vi "PreferenceFolder.vi"() -> (0 "error out":errorcluster, 1 "Colors":u32[](array[numeric]), 2 "FontSize":u8, 3 "pythonCodes":path[](array[path]), 4 "SSH Logins":T3(array[cluster]), 5 "Examples":path, 6 "Pis":T2(array[cluster]), 7 "Everything":T1={"python"="", "arduino CLI"=path "", "pythonCodes"=[], "FontSize"=0, "Text Colors"={"Quote"=46086, "function"=239, "Python"=11817216, "Comment"=15665920, "Triple Quote"=9306312, "Text"=0}, "SSH Logins"=[], "packet size"=32})   [LabVIEW 2024]
uses:
  Preferences.ctl
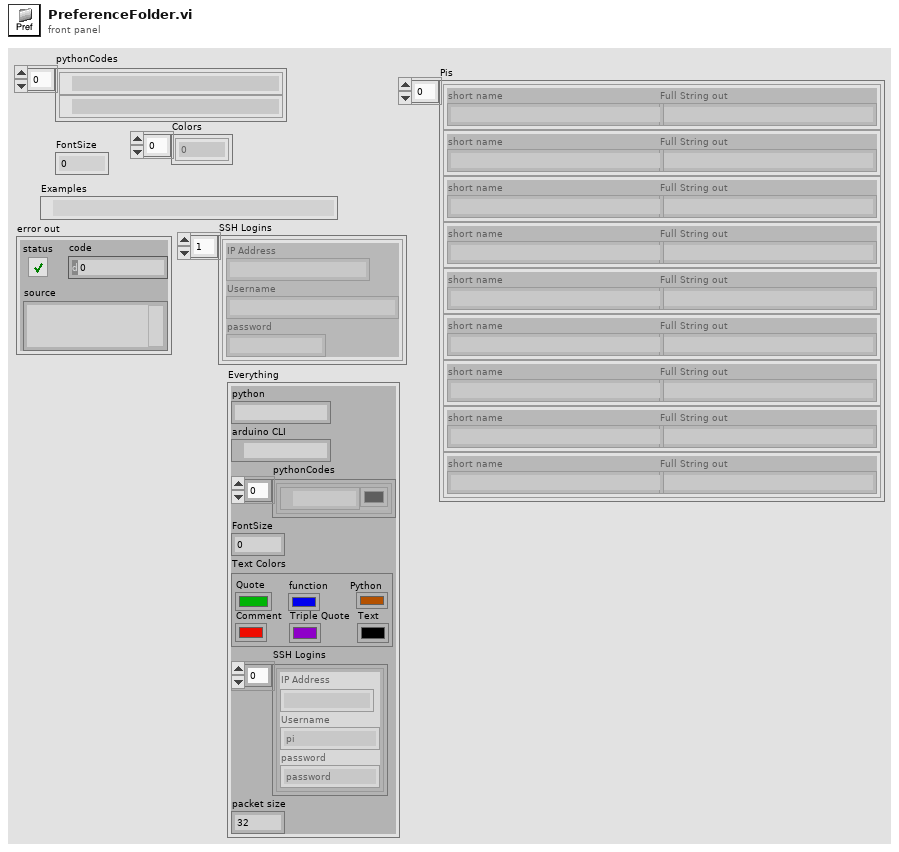
[diagram p1: front panel]
types:
  T1 = typedef "Preferences.ctl" = cluster{"python":string, "arduino CLI":path, "pythonCodes":cluster{"pythonCode":path, "Color":u32}[], "FontSize":u8, "Text Colors":cluster{"Quote":u32, "function":u32, "Python":u32, "Comment":u32, "Triple Quote":u32, "Text":u32}, "SSH Logins":cluster{"IP Address":string, "Username":string, "password":string}[], "packet size":u8}
  T2 = cluster{"short name":string, "Full String out":string}[]
  T3 = cluster{"IP Address":string, "Username":string, "password":string}[]
  T4 = cluster{"short name":string, "Full String out":string}
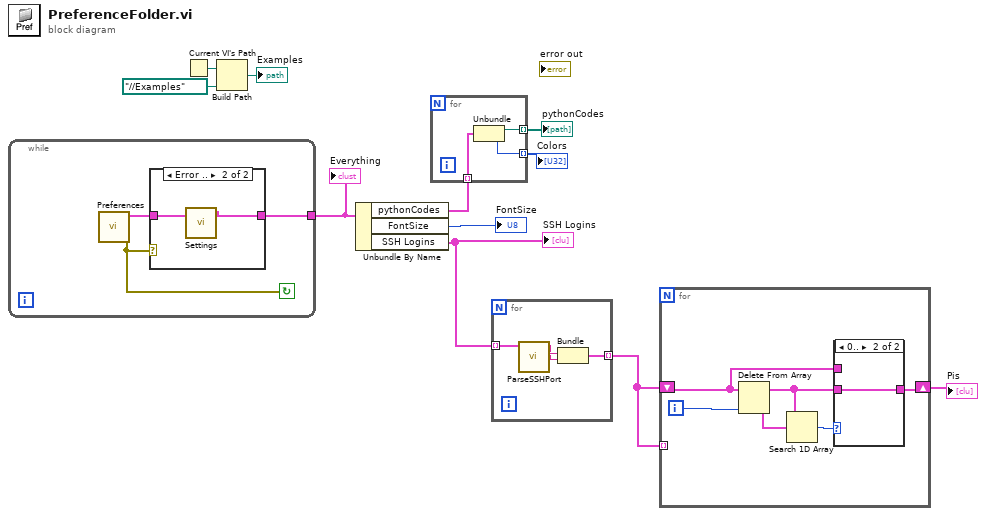
[diagram p0: block diagram]
diagram:
  n1 = while {
    tunnel: [w12] -> w10
    stop <- w14 continue-if-true
    n2 = call "Preferences.vi"() -> ("error out"=w14:errorcluster, "Preferences out"=w13:T1)  [unwired: 10 in]
    n3 = case shown="Error .." w14 {
      tunnel: w13 -> [w15 w17]
      tunnel: [w15 w16] -> w12
      frame No Error {
      }
      frame Error {
        n4 = call "Settings.vi"("Prefs"=w17) -> ("Preferences"=w16:T1)  [unwired: 10 in]
      }
    }
  }
  "Everything" <- w10
  n5 = Current VI's Path() -> (path=w6:path)
  n6 = Build Path(base path=w6, name or relative path=path "../../Examples") -> (appended path=→"Examples":path)
  n7 = Unbundle By Name(w10) -> ("pythonCodes"=w9:cluster{"pythonCode":path, "Color":u32}[], "FontSize"=→"FontSize":u8, "SSH Logins"=w3:T3)
  "SSH Logins" <- w3
  n8 = for {
    tunnel: w9 -> [w20] mode=indexing
    tunnel: [w19] -> w8 mode=indexing
    tunnel: [w18] -> w7 mode=indexing
    n9 = Unbundle(w20) -> ("pythonCode"=w19:path, "Color"=w18:u32)
  }
  "pythonCodes" <- w8
  "Colors" <- w7
  n10 = for {
    tunnel: w3 -> [w24] mode=indexing
    tunnel: [w21] -> w2 mode=indexing
    n11 = call "ParseSSHPort.vi"("SSH Login"=w24) -> ("short name"=w23:string, "Full String out"=w22:string)  [unwired: 8 in, 1 out]
    n12 = Bundle("short name"=w23, "Full String out"=w22) -> (w21:T4)  [unwired: 1 in]
  }
  n13 = for {
    tunnel: w2 -> [_] mode=indexing
    shift-right: [w28] -> w1
    shift-left: w2 -> [w26]
    i -> [w30]
    n14 = Delete From Array(array=w26, index=w30) -> (deleted portion=w29:T4, array with subset deleted=w25:T2)  [unwired: 1 in]
    n15 = Search 1D Array(1D array=w25, element=w29) -> (index of element=w27:i32)  [unwired: 1 in]
    n16 = case shown="0.." w27 {
      tunnel: w26 -> [w31 _]
      tunnel: [w31 w32] -> w28
      tunnel: w25 -> [_ w32]
      frame ..-1 {
      }
      frame 0.. {
      }
    }
  }
  "Pis" <- w1
